vi "FL_DEC_split_array.vi"(2 "Input DEC array":sgl[][](array[numeric])) -> (0 "ms since ON":u32[](array[numeric]), 1 "Channel":u32[](array[numeric]), 3 "delta time":u32[](array[numeric]), 4 "Err. lenght":dbl[](array[numeric]), 5 "TTL input 1":sgl[](array[numeric]), 6 "X1":sgl[](array[numeric]), 7 "Y1":sgl[](array[numeric]), 8 "TTL input 2":sgl[](array[numeric]), 9 "X2":sgl[](array[numeric]), 10 "Y2":sgl[](array[numeric]))   [LabVIEW 2016]
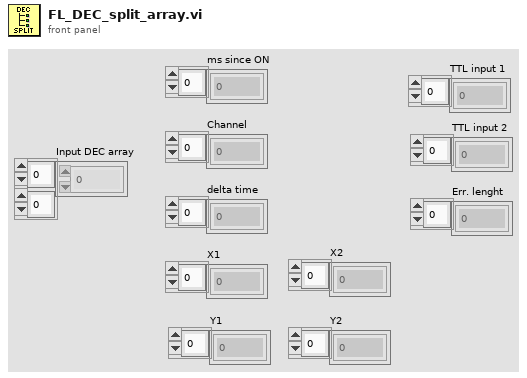
[diagram p1: front panel]
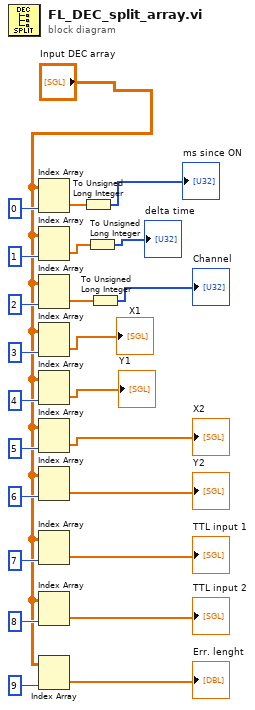
[diagram p0: block diagram]
diagram:
  n1 = Index Array(array="Input DEC array", index (col)=0 ("disabled index (col)")) -> (element=w13:sgl[])  [unwired: 1 in]
  n2 = Index Array(array="Input DEC array", index (col)=1 ("disabled index (col)")) -> (element=w11:sgl[])  [unwired: 1 in]
  n3 = Index Array(array="Input DEC array", index (col)=2 ("disabled index (col)")) -> (element=w10:sgl[])  [unwired: 1 in]
  n4 = Index Array(array="Input DEC array", index (col)=3 ("disabled index (col)")) -> (element=→"X1":sgl[])  [unwired: 1 in]
  n5 = Index Array(array="Input DEC array", index (col)=4 ("disabled index (col)")) -> (element=→"Y1":sgl[])  [unwired: 1 in]
  n6 = Index Array(array="Input DEC array", index (col)=5 ("disabled index (col)")) -> (element=→"X2":sgl[])  [unwired: 1 in]
  n7 = Index Array(array="Input DEC array", index (col)=6 ("disabled index (col)")) -> (element=→"Y2":sgl[])  [unwired: 1 in]
  n8 = Index Array(array="Input DEC array", index (col)=7 ("disabled index (col)")) -> (element=→"TTL input 1":sgl[])  [unwired: 1 in]
  n9 = Index Array(array="Input DEC array", index (col)=8 ("disabled index (col)")) -> (element=→"TTL input 2":sgl[])  [unwired: 1 in]
  n10 = Index Array(array="Input DEC array", index (col)=9 ("disabled index (col)")) -> (element=→"Err. lenght":sgl[])  [unwired: 1 in]
  n11 = To Unsigned Long Integer(number=w13) -> (unsigned 32bit integer=→"ms since ON":u32[])
  n12 = To Unsigned Long Integer(number=w11) -> (unsigned 32bit integer=→"delta time":u32[])
  n13 = To Unsigned Long Integer(number=w10) -> (unsigned 32bit integer=→"Channel":u32[])
